vi "Graphics-Set Line Styles.vi"(0 "XY Graph":refnum<vi>, 1 "Max Ncolor":i32, 2 "Map":T1(ring), 5 "Colors":u32[](array[colorbox]), 7 "Plot.Line Width":u8=1, 9 "Plot.Point Style":u8, 11 "error in (no error)":errorcluster) -> (4 "XY Graph out":refnum<vi>, 15 "error out":errorcluster)   [LabVIEW 2020]
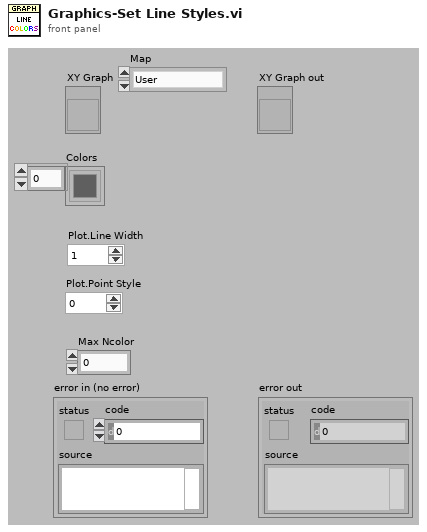
[diagram p1: front panel]
types:
  T1 = enum16{"User", "Prism", "Kelly", "Dark2", "Sequential", "Hue"}
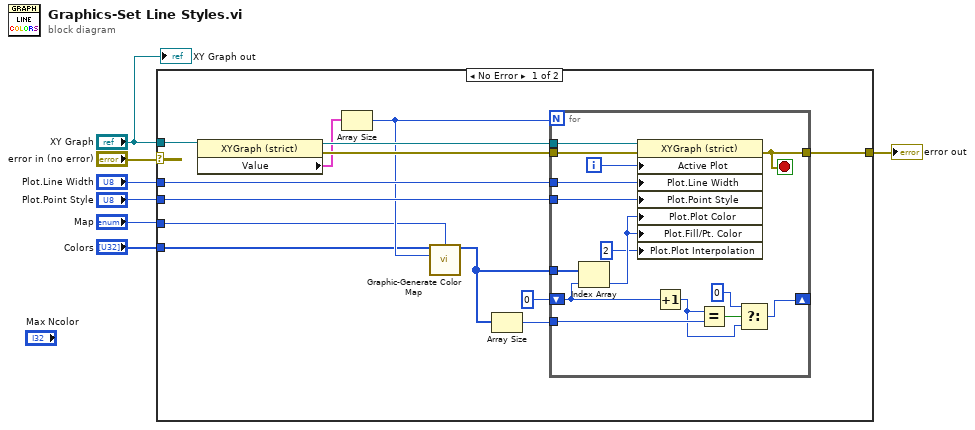
[diagram p0: block diagram]
diagram:
  n1 = case shown="No Error" "error in (no error)" {
    selector: "error in (no error)" -> [_ w36]
    tunnel: "XY Graph" -> [w20 _]
    tunnel: "Colors" -> [w10 _]
    tunnel: [w16 w36] -> w4
    tunnel: "Plot.Line Width" -> [w15 _]
    tunnel: "Map" -> [w8 _]
    tunnel: "Plot.Point Style" -> [w12 _]
    frame No Error {
      n2 = property class="XYGraph (strict)"(reference=w20) -> (reference out=w19:refnum<vi>, error out=w18:errorcluster, "Value"=w17:cluster{"Frequency":dbl[], "Frequency":dbl[]}[])  [unwired: 1 in]
      n3 = Array Size(array=w17) -> (size(s)=w11:i32)
      n4 = call "Graphic-Generate Color Map.vi"("User"=w10, "Map"=w8, "Size"=w11) -> ("Colors"=w9:u32[])  [unwired: 12 in]
      n5 = Array Size(array=w9) -> (size(s)=w13:i32)
      n6 = for {
        N: w11 -> [_]
        tunnel: w19 -> [w35]
        tunnel: w18 -> [w34]
        tunnel: [w32] -> w16
        tunnel: w15 -> [w31]
        shift-right: [w24] -> _
        shift-left: 0 -> [w29]
        tunnel: w9 -> [w30]
        tunnel: w13 -> [w28]
        tunnel: w12 -> [w23]
        i -> [w33]
        stop <- w32 stop-if-true
        n7 = Index Array(array=w30, index=w29) -> (element=w22:u32)
        n8 = property class="XYGraph (strict)"(reference=w35, error in=w34, "Active Plot"=w33, "Plot.Line Width"=w31, "Plot.Point Style"=w23, "Plot.Plot Color"=w22, "Plot.Fill/Pt. Color"=w22, "Plot.Plot Interpolation"=u8 2) -> (error out=w32:errorcluster)  [unwired: 1 out]
        n9 = Increment(x=w29) -> (x+1=w26:i32)
        n10 = Equal?(x=w26, y=w28) -> (x = y?=w27:bool)
        n11 = Select(t=0, s=w27, f=w26) -> (s? t:f=w24:i32)
      }
    }
    frame Error {
    }
  }
  "error out" <- w4
  "XY Graph out" <- "XY Graph"
